vi "Stop Core.vi"(10 "final error code":i32, 11 "Command in":refnum<class "Command.lvclass">) -> (3 "Command out":refnum<class "Command.lvclass">)   [LabVIEW 2013, in "Robot Actors.lvlib" / "Command.lvlib" / "Command.lvclass"]
doc: "(<B>Filename</B>: Actor Framework.lvlib:Actor.lvclass:Stop Core.vi)\n\nDefines what the actor does before it stops. Use the <B>final error code</B> input to determine whether the actor shut down in response to an error.\n\nBy default, this method does nothing. A descendant class may override it to define behavior, such as shutting down any processes the actor initiated in its override of the Actor Core method."
uses:
  Command.lvclass
  State Actor/State Actor.lvclass
  Command.lvclass/Command.ctl
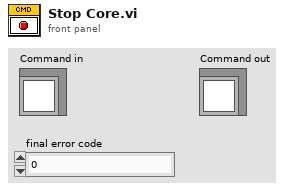
[diagram p1: front panel]
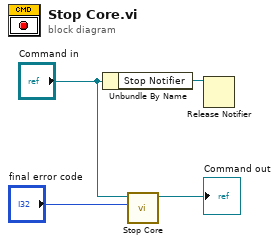
[diagram p0: block diagram]
diagram:
  n1 = Unbundle By Name("Command in") -> ("Stop Notifier"=w2:refnum<notifier>)
  n2 = call-parent "Stop Core.vi"("final error code"="final error code", "Actor in"="Command in") -> ("Actor out"=→"Command out":refnum<class "Command.lvclass">)  [unwired: 9 in]
  n3 = Release Notifier(notifier=w2) -> ()  [unwired: 2 in, 3 out]
